vi "Query Trace Fail.vi"(8 "error in (no error)":errorcluster {"code" format="%.0x"}, 9 "DigitalDemodWindow":string="Window1\nAverageMode\nAverageMode", 11 "instrument handle":refnum<k15>) -> (0 "error out":errorcluster {"code" format="%.0x"}, 2 "Val":bool, 3 "instrument handle out":refnum<k15>)   [LabVIEW 2021, in "Keysight XSAnVMA.lvlib"]
doc: "Tests the trace in the window against all associated limit lines."
uses:
  <instrlib>/Keysight XSAnVMA/Keysight XSAnVMA.lvlib
  KtXSAnVMA_64.dll
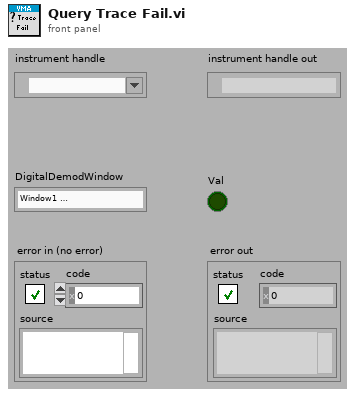
[diagram p1: front panel]
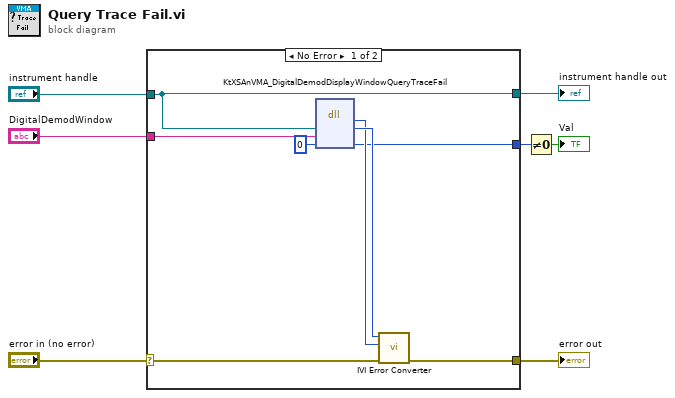
[diagram p0: block diagram]
diagram:
  n1 = case shown="No Error" "error in (no error)" {
    selector: "error in (no error)" -> [w13 w17]
    tunnel: [w12 w17] -> w7
    tunnel: "instrument handle" -> [w8 w16]
    tunnel: "DigitalDemodWindow" -> [w11 _]
    tunnel: [w9 _] -> w2
    tunnel: [w8 w16] -> w1
    frame No Error {
      n2 = dll-call lib="KtXSAnVMA**.dll" fn="KtXSAnVMA_DigitalDemodDisplayWindowQueryTraceFail"("Vi"=w8, "DigitalDemodWindow"=w11, "Val"=i16 0) -> (w14:i32, "Vi"=w15:u32, "Val"=w9:i16)  [unwired: 4 in, 2 out]
      n3 = call <instrlib>:"IVI Error Converter.vi"("error in (no error)"=w13, "IVI error code (0)"=w14, "instrument handle"=w15) -> ("error out"=w12:errorcluster)  [unwired: 7 in, 1 out]
    }
    frame Error {
    }
  }
  "error out" <- w7
  "instrument handle out" <- w1
  n4 = Not Equal To 0?(x=w2) -> (x != 0?=→"Val":bool)
